vi "Config Panel.vi"(7 "Error In":errorcluster, 10 "MSX-E3701 in":refnum<class "MSX-E3701.lvclass">) -> (0 "Error Out":errorcluster, 3 "MSX-E3701 out":refnum<class "MSX-E3701.lvclass">)   [LabVIEW 2014, in "MSX-E3701.lvlib" / "MSX-E3701.lvclass"]
doc: "PANEL FRONTAL PARA PRICIPAL DE CONFIGURACION."
uses:
  MSX-E3701Class/MSX-E3701.lvclass
  MSX-E3701Class/MSX-E3701.lvclass/MSX-E3701.ctl
  API/MSX-E3701_dll.lvlib
  DriverMasterSync/build/DriverMasterSync.lvlibp/Modules/HAL/DriverMasterSync/DriverMasterSyncClass/DriverMasterSync.lvclass
panel:
  in  "Aplicar":bool
  in  "Cancelar":bool
  in  "Aceptar":bool
  in  "DIO Enable":bool=TRUE
  in  "Protection":bool
  in  "Transducer Selection":bool
  in  "Offset":bool
  in  "Gain":bool
  in  "Diagnostic":bool
  in  "Calibration":bool
  in  "Transductores":bool[][](array[boolean])
  in  "Division Factor":u64=5
  in  "Nbr Of Sequence":u64
  in  "Nbr Max Sequence To Transfer":u64=800
  in  "Division Factor":u64=5
  in  "Connection Data.IP":string="192.168.99.99"
  # "ADDI-DATA MSX-E3701"
  # "IP Config"
  # "Sequence"
  # "AutoRefresh"
  # "1"
  # "2"
  # "3"
  # "4"
  # "5"
  # "6"
  # "7"
  # "8"
  # "9"
  # "10"
  # "11"
  # "12"
  # "13"
  # "14"
  # "15"
  # "16"
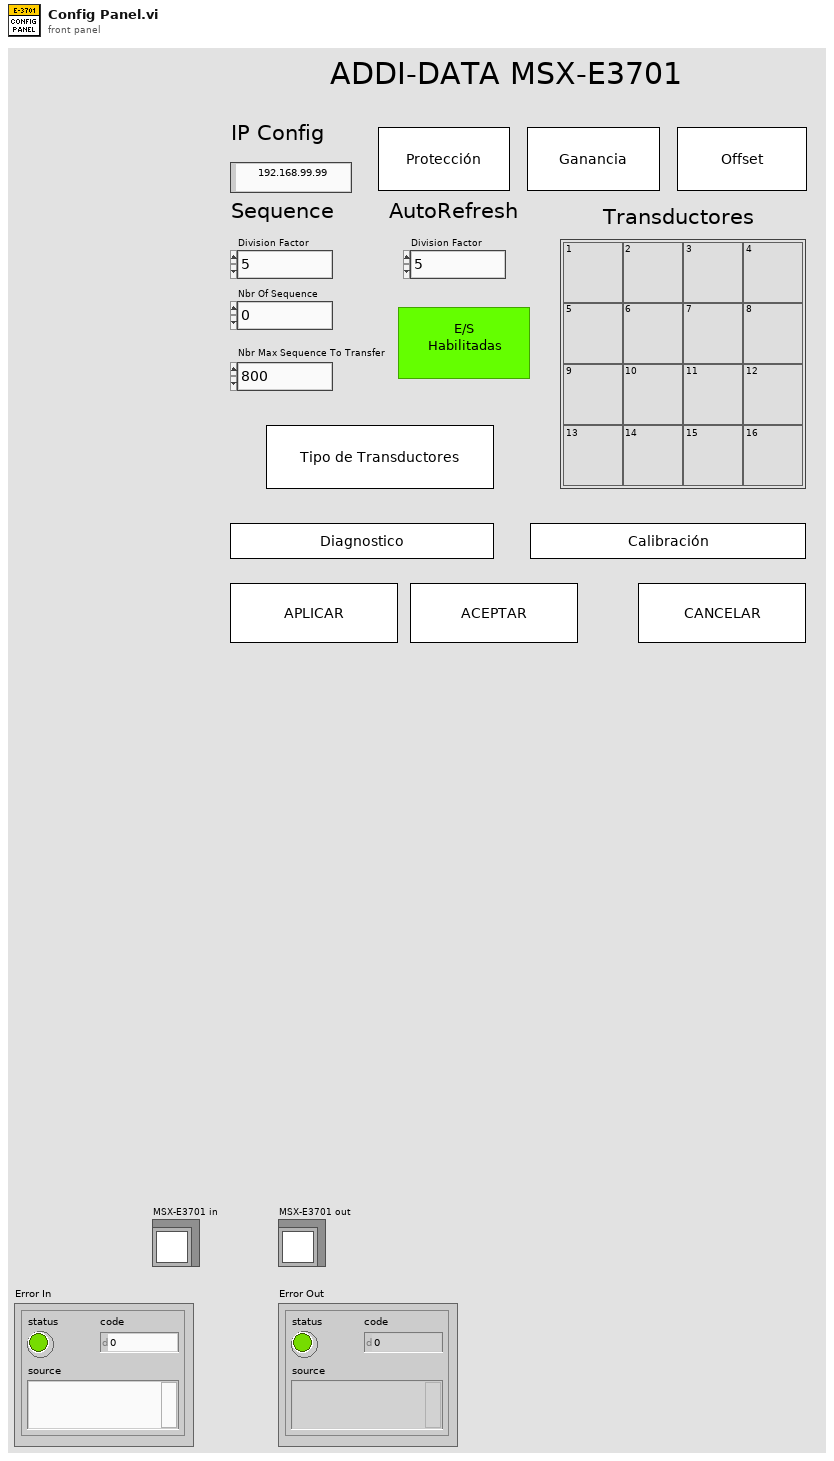
[diagram p1: front panel]
types:
  T1 = typedef "DriverMasterSync.lvlibp/HAL Config Data.ctl" = cluster{"HWSync Index":u32, "Driver Name":string, "Channel Mask":u64}
  T2 = typedef "MSX-E3701_dll.lvlib/Config Data.ctl" = cluster{"Auto Refresh":cluster{"Average Mode":u64, "Average Value":u64, "Division Factor":u64, "Trigger Action":u64, "Hardware Trigger Count":u64, "Hardware Trigger Filter Time":u64, "By Trigger Nbr Of Seq To Acquire":u64, "Time stamp":bool, "Analog Output(mm)":bool, "Invert value":bool}, "Gain":sgl[], "Offset":sgl[], "Index":u64, "Range":sgl, "Sequence":cluster{"Division Factor":u64, "Nbr Of Sequence":u64, "Nbr Max Sequence To Transfer":u64, "Sequence.Delay Mode":u64, "Delay Time Unit":u64, "Delay Value":u64, "Trigger Action":u64, "Hardware Trigger Count":u64, "Hardware Trigger Filter Time":u64, "By Trigger Nbr Of Seq To Acquire":u64, "Time stamp":bool, "Sequence counter information":bool, "Analog Output(mm)":bool, "Invert value":bool, "Relative Time Stamp":bool, "Hardware trigger information":bool}, "Enable DIO":bool}
  T3 = cluster{"Average Mode":u64, "Average Value":u64, "Division Factor":u64, "Trigger Action":u64, "Hardware Trigger Count":u64, "Hardware Trigger Filter Time":u64, "By Trigger Nbr Of Seq To Acquire":u64, "Time stamp":bool, "Analog Output(mm)":bool, "Invert value":bool}
  T4 = cluster{"Division Factor":u64, "Nbr Of Sequence":u64, "Nbr Max Sequence To Transfer":u64, "Sequence.Delay Mode":u64, "Delay Time Unit":u64, "Delay Value":u64, "Trigger Action":u64, "Hardware Trigger Count":u64, "Hardware Trigger Filter Time":u64, "By Trigger Nbr Of Seq To Acquire":u64, "Time stamp":bool, "Sequence counter information":bool, "Analog Output(mm)":bool, "Invert value":bool, "Relative Time Stamp":bool, "Hardware trigger information":bool}
  T5 = typedef "MSX-E3701_dll.lvlib/Connection Data.ctl" = cluster{"MX370x refnum":refnum<k24>, "IP":string, "Connection ID ":refnum<k5>, "MXCommon refnum":refnum<k24>}
  T6 = typedef "MSX-E3701_dll.lvlib/Diagnostic Data.ctl" = cluster{"Muestras Diag. Cycle":u32, "Tolerancia Cycle":sgl, "Tolerancia":sgl, "Mask Proteccion T":u64, "Promedio Transd":sgl[]}
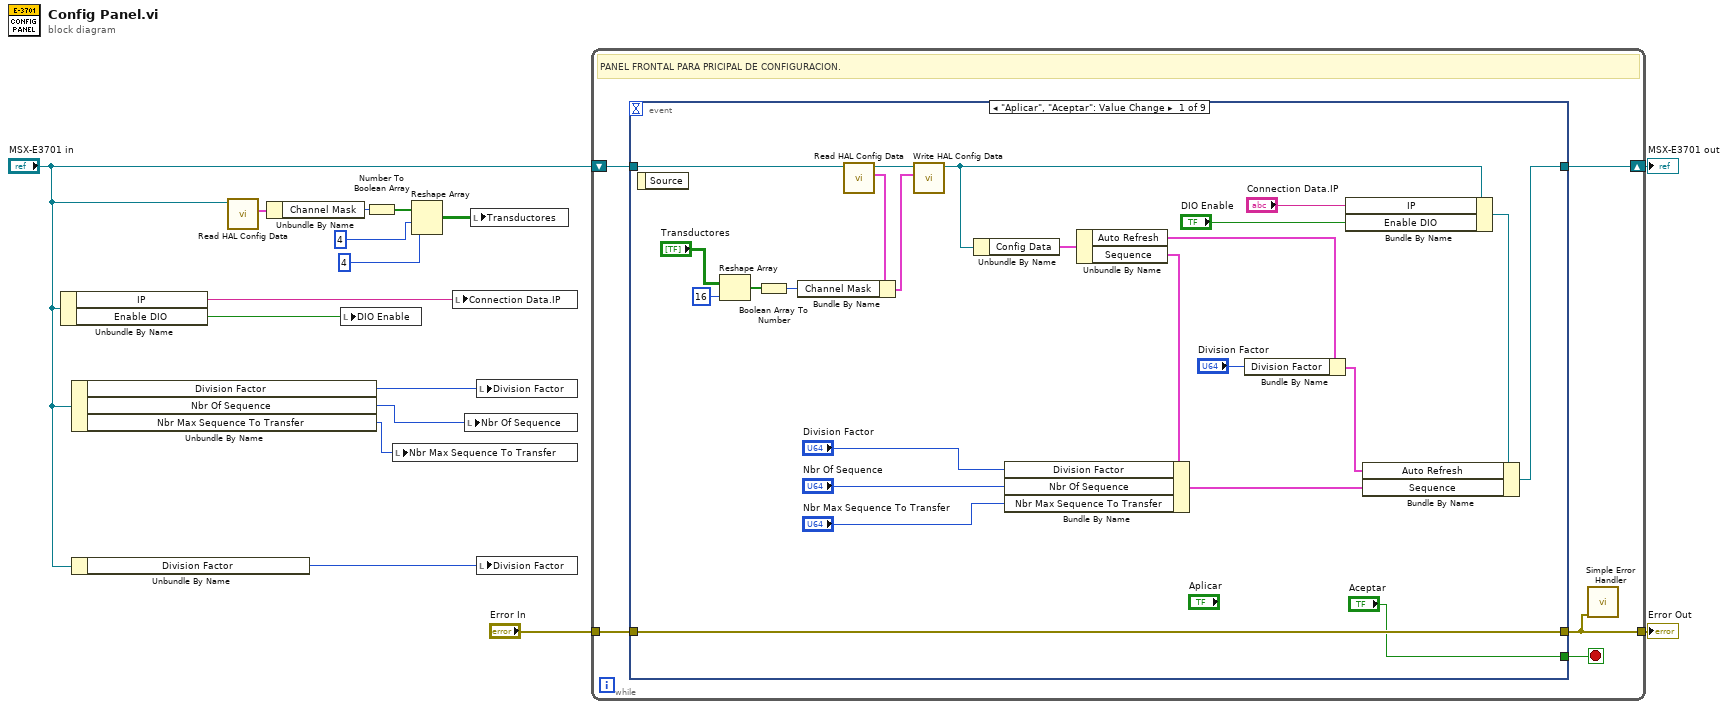
[diagram p0: block diagram]
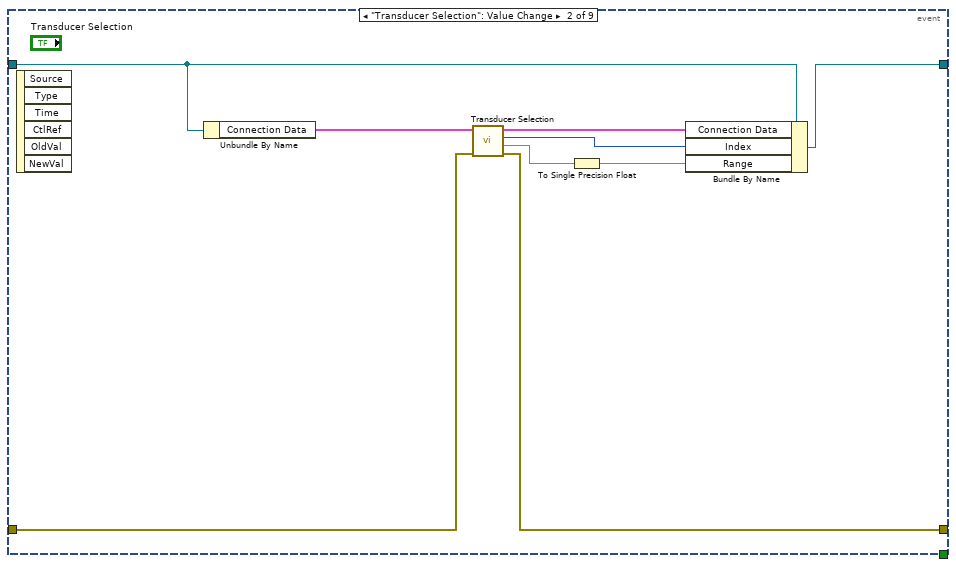
[diagram p2: hidden frame]
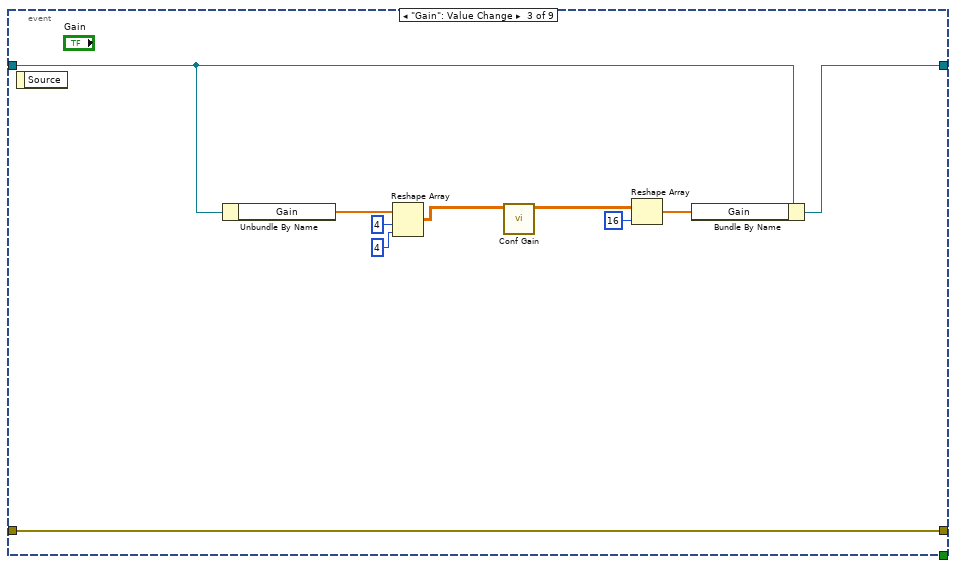
[diagram p3: hidden frame]
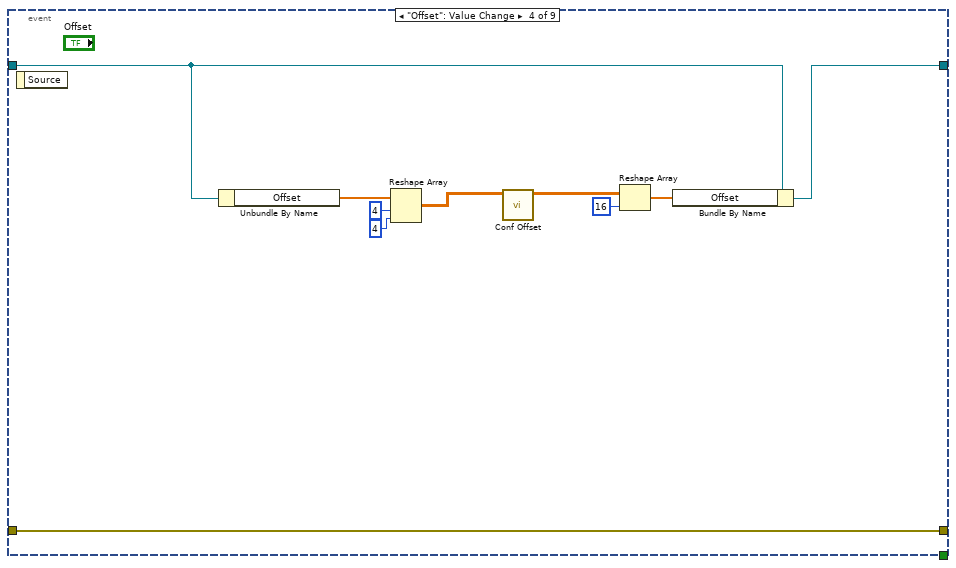
[diagram p4: hidden frame]
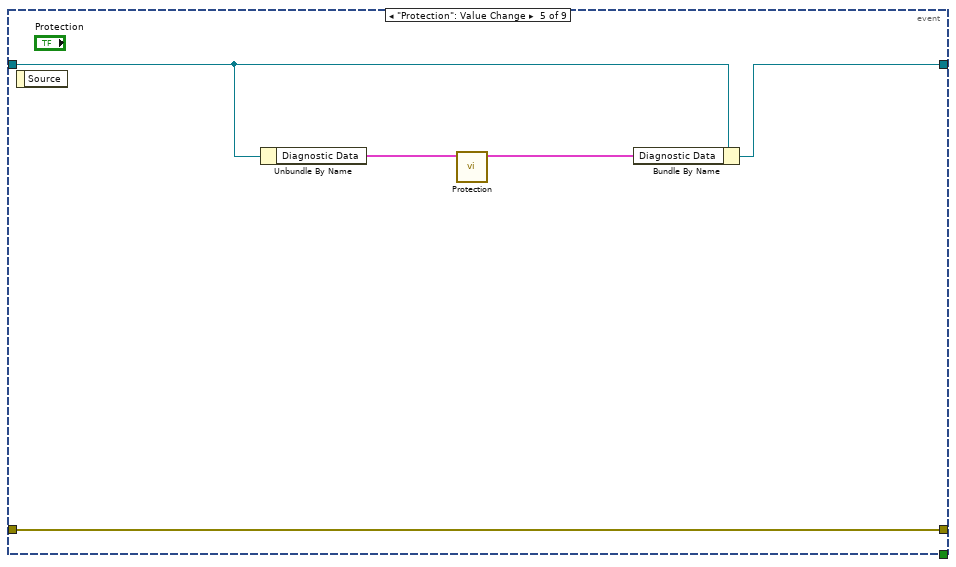
[diagram p5: hidden frame]
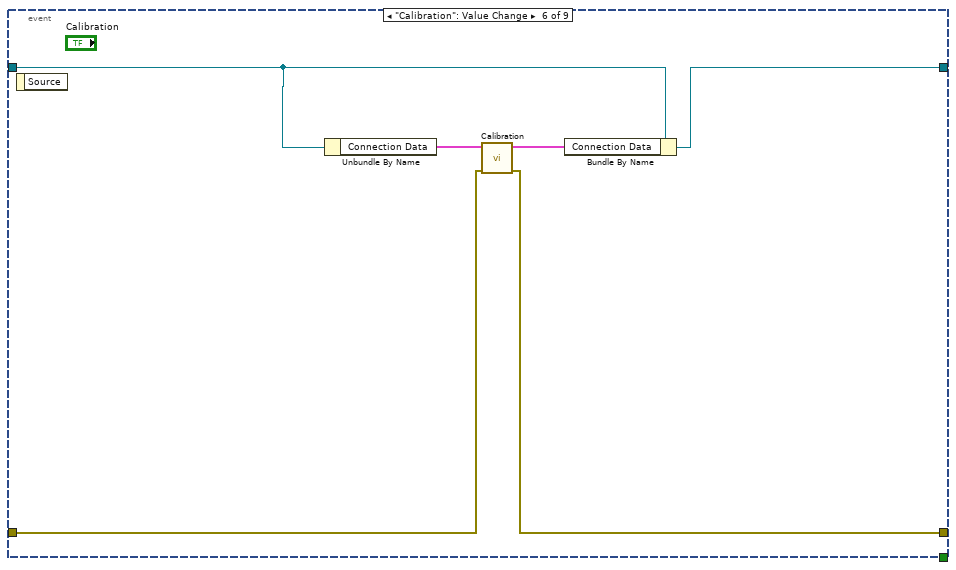
[diagram p6: hidden frame]
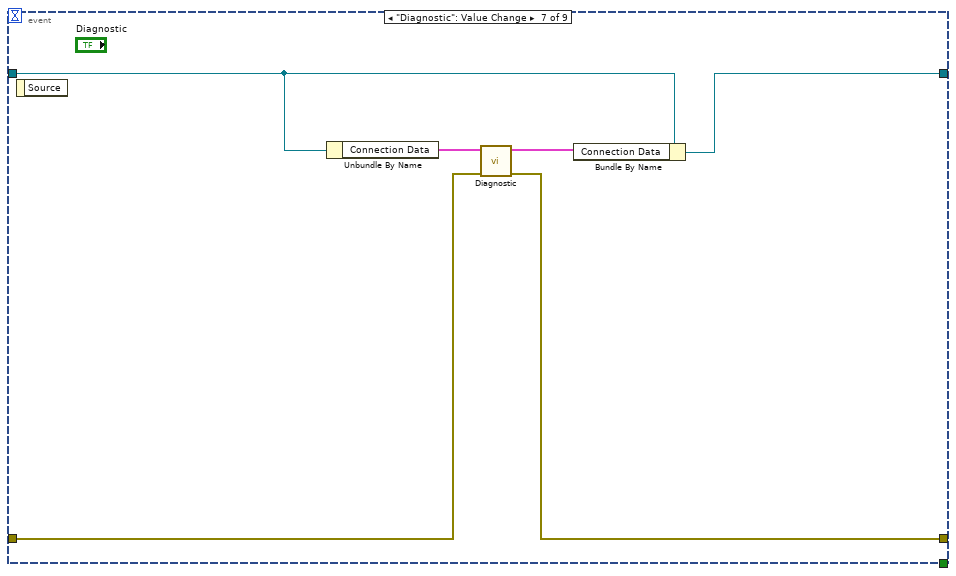
[diagram p7: hidden frame]
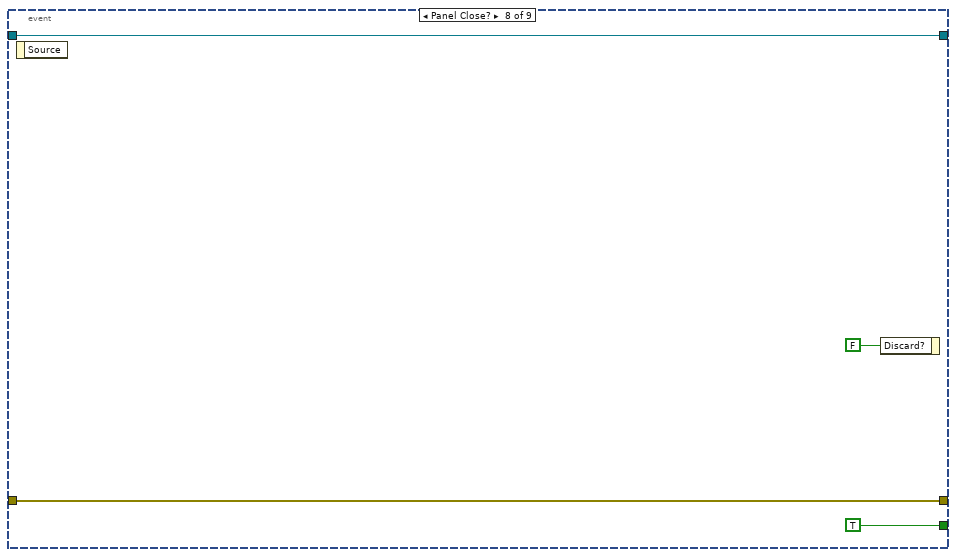
[diagram p8: hidden frame]
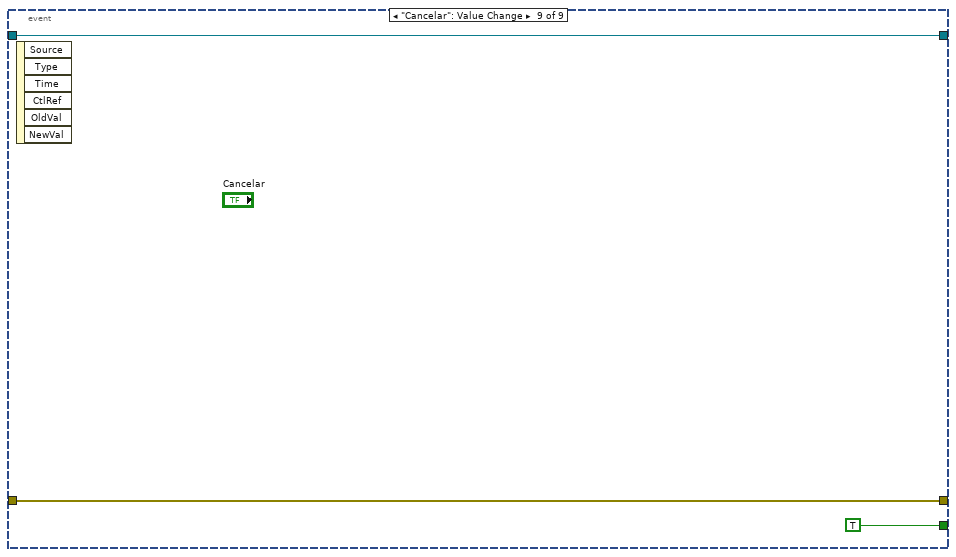
[diagram p9: hidden frame]
diagram:
  n1 = Unbundle By Name("MSX-E3701 in") -> ("IP"=w2:string, "Enable DIO"=w1:bool)
  n2 = Unbundle By Name("MSX-E3701 in") -> ("Division Factor"=w7:u64, "Nbr Of Sequence"=w6:u64, "Nbr Max Sequence To Transfer"=w5:u64)
  n3 = Unbundle By Name("MSX-E3701 in") -> ("Division Factor"=w4:u64)
  n4 = call "Read HAL Config Data.vi"("DriverMasterSync in"="MSX-E3701 in") -> ("HAL Config Data"=w13:T1)  [unwired: 8 in, 2 out]
  n5 = Unbundle By Name(w13) -> ("Channel Mask"=w12:u64)
  n6 = local write "DIO Enable"(w1) -> ()
  n7 = Number To Boolean Array(number=w12) -> (Boolean array=w11:bool[])
  n8 = local write "Nbr Max Sequence To Transfer"(w5) -> ()
  n9 = Reshape Array(w11, 4 ("dimension size"), 4 ("dimension size")) -> (w10:bool[][])
  n10 = local write "Connection Data.IP"(w2) -> ()
  n11 = local write "Nbr Of Sequence"(w6) -> ()
  n12 = local write "Transductores"(w10) -> ()
  n13 = local write "Division Factor"(w7) -> ()
  n14 = local write "Division Factor"(w4) -> ()
  n15 = while {
    tunnel: [w18] -> w15
    tunnel: "Error In" -> [w19]
    shift-right: [w17] -> w16
    shift-left: "MSX-E3701 in" -> [w20]
    stop <- w21 stop-if-true
    # "PANEL FRONTAL PARA PRICIPAL DE CONFIGURACION."
    n16 = event shown="[0] \"Aplicar\", \"Aceptar\": Value Change" {
      selector: _ -> [_ _ _ _ _ _ _ _ _]
      dyn-events: _ -> [_ _ _ _ _ _ _ _ _]
      timeout: _ -> [_ _ _ _ _ _ _ _ _]
      tunnel: ["Aceptar" _ _ _ _ _ _ TRUE ("Cancel Program") TRUE ("Cancel Program")] -> w21
      tunnel: [w43 w53 w62 w72 w75 w83 w88 w95 w98] -> w17
      tunnel: w20 -> [w27 w54 w63 w73 w76 w80 w89 w95 w98]
      tunnel: w19 -> [w33 w48 w64 w74 w79 w82 w87 w94 w97]
      tunnel: [w33 w49 w64 w74 w79 w81 w86 w94 w97] -> w18
      event "Aplicar", "Aceptar": Value Change {
        n17 = event-data() -> ()  [unwired: 1 in, 1 out]
        n18 = Reshape Array("Transductores", 16 ("dimension size")) -> (w32:bool[])
        n19 = Boolean Array To Number(Boolean array=w32) -> (number=w25:u64)
        n20 = call "Read HAL Config Data.vi"("DriverMasterSync in"=w27) -> ("HAL Config Data"=w29:T1, "DriverMasterSync out"=w30:refnum<class "MSX-E3701.lvclass">)  [unwired: 8 in, 1 out]
        n21 = Bundle By Name(cluster=w29, "Channel Mask"=w25) -> (w28:T1)
        n22 = call "Write HAL Config Data.vi"("HAL Config Data"=w28, "DriverMasterSync in"=w30) -> ("DriverMasterSync out"=w26:refnum<class "MSX-E3701.lvclass">)  [unwired: 8 in, 1 out]
        n23 = Unbundle By Name(w26) -> ("Config Data"=w44:T2)
        n24 = Unbundle By Name(w44) -> ("Auto Refresh"=w37:T3, "Sequence"=w38:T4)
        n25 = Bundle By Name(cluster=w38, "Division Factor"="Division Factor", "Nbr Of Sequence"="Nbr Of Sequence", "Nbr Max Sequence To Transfer"="Nbr Max Sequence To Transfer") -> (w35:T4)
        n26 = Bundle By Name(cluster=w37, "Division Factor"="Division Factor") -> (w34:T3)
        n27 = Bundle By Name(cluster=w26, "IP"="Connection Data.IP", "Enable DIO"="DIO Enable") -> (w42:refnum<class "MSX-E3701.lvclass">)
        n28 = Bundle By Name(cluster=w42, "Auto Refresh"=w34, "Sequence"=w35) -> (w43:refnum<class "MSX-E3701.lvclass">)
      }
      event "Transducer Selection": Value Change {
        n29 = event-data() -> ()  [unwired: 1 in, 6 out]
        n30 = Unbundle By Name(w54) -> ("Connection Data"=w52:T5)
        n31 = call "Transducer Selection.vi"("error in (no error)"=w48, "Connection Data In"=w52) -> ("error out"=w49:errorcluster, "Range"=w47:dbl, "Index"=w50:u64, "Connection Data Out"=w51:T5)  [unwired: 5 in]
        n32 = To Single Precision Float(number=w47) -> (single precision float=w46:sgl)
        n33 = Bundle By Name(cluster=w54, "Connection Data"=w51, "Index"=w50, "Range"=w46) -> (w53:refnum<class "MSX-E3701.lvclass">)
      }
      event "Gain": Value Change {
        n34 = event-data() -> ()  [unwired: 1 in, 1 out]
        n35 = Unbundle By Name(w63) -> ("Gain"=w61:sgl[])
        n36 = Reshape Array(w61, 4 ("dimension size"), 4 ("dimension size")) -> (w60:sgl[][])
        n37 = call "Conf Gain.vi"("Gain in"=w60) -> ("Gain Out"=w57:sgl[][])  [unwired: 10 in]
        n38 = Reshape Array(w57, 16 ("dimension size")) -> (w55:sgl[])
        n39 = Bundle By Name(cluster=w63, "Gain"=w55) -> (w62:refnum<class "MSX-E3701.lvclass">)
      }
      event "Offset": Value Change {
        n40 = event-data() -> ()  [unwired: 1 in, 1 out]
        n41 = Unbundle By Name(w73) -> ("Offset"=w68:sgl[])
        n42 = Reshape Array(w68, 4 ("dimension size"), 4 ("dimension size")) -> (w67:sgl[][])
        n43 = call "Conf Offset.vi"("Offset in"=w67) -> ("Offset Out"=w66:sgl[][])  [unwired: 10 in]
        n44 = Reshape Array(w66, 16 ("dimension size")) -> (w65:sgl[])
        n45 = Bundle By Name(cluster=w73, "Offset"=w65) -> (w72:refnum<class "MSX-E3701.lvclass">)
      }
      event "Protection": Value Change {
        n46 = event-data() -> ()  [unwired: 1 in, 1 out]
        n47 = Unbundle By Name(w76) -> ("Diagnostic Data"=w78:T6)
        n48 = call "Protection.vi"("Diagnostic Data"=w78) -> ("Diagnostic Data out"=w77:T6)  [unwired: 10 in]
        n49 = Bundle By Name(cluster=w76, "Diagnostic Data"=w77) -> (w75:refnum<class "MSX-E3701.lvclass">)
      }
      event "Calibration": Value Change {
        n50 = event-data() -> ()  [unwired: 1 in, 1 out]
        n51 = Unbundle By Name(w80) -> ("Connection Data"=w84:T5)
        n52 = call "Calibration.vi"("error in (no error)"=w82, "Connection Data In"=w84) -> ("error out"=w81:errorcluster, "Connection Data Out"=w85:T5)  [unwired: 8 in]
        n53 = Bundle By Name(cluster=w80, "Connection Data"=w85) -> (w83:refnum<class "MSX-E3701.lvclass">)
      }
      event "Diagnostic": Value Change {
        n54 = event-data() -> ()  [unwired: 1 in, 1 out]
        n55 = Unbundle By Name(w89) -> ("Connection Data"=w91:T5)
        n56 = call "Diagnostic.vi"("error in (no error)"=w87, "Connection Data In"=w91) -> ("error out"=w86:errorcluster, "Connection Data Out"=w90:T5)  [unwired: 8 in]
        n57 = Bundle By Name(cluster=w89, "Connection Data"=w90) -> (w88:refnum<class "MSX-E3701.lvclass">)
      }
      event Panel Close? {
        n58 = event-data() -> ()  [unwired: 1 in, 1 out]
        n59 = event-data("Discard?"=FALSE) -> ()  [unwired: 1 in, 1 out]
      }
      event "Cancelar": Value Change {
        n60 = event-data() -> ()  [unwired: 1 in, 6 out]
      }
    }
    n61 = call <vilib>:"Simple Error Handler.vi"("error in (no error)"=w18) -> ()  [unwired: 4 in, 5 out]
  }
  "MSX-E3701 out" <- w16
  "Error Out" <- w15
